vi "Rename Node Name.vi"(8 "error in (no error)":errorcluster, 10 "Node Tag":string, 11 "TREE in":refnum<class "MyTreeAPI.lvclass">) -> (0 "error out":errorcluster, 3 "TREE out":refnum<class "MyTreeAPI.lvclass">)   [LabVIEW 2015, in "MyTreeAPI.lvclass"]
uses:
  MyTreeAPI.lvclass
  MyTreeAPI.lvclass/MyTreeAPI.ctl
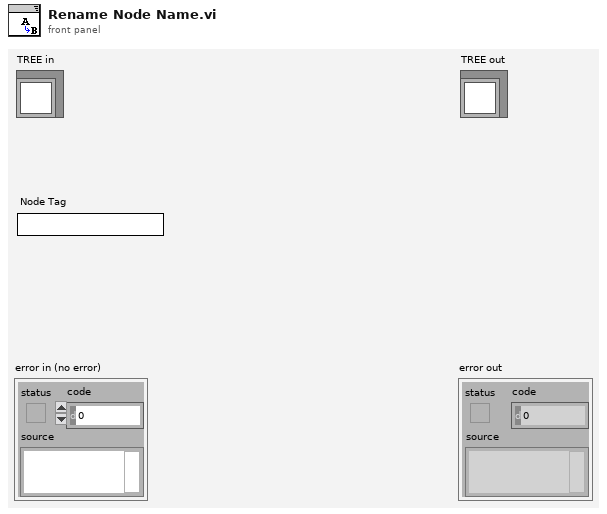
[diagram p1: front panel]
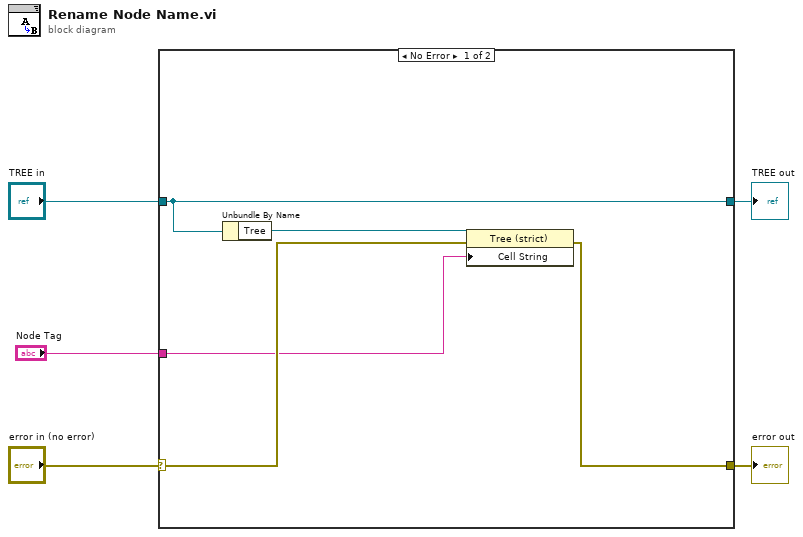
[diagram p0: block diagram]
diagram:
  n1 = case shown="No Error" "error in (no error)" {
    selector: "error in (no error)" -> [w8 w12]
    tunnel: [w6 w12] -> w4
    tunnel: [w10 w11] -> w2
    tunnel: "TREE in" -> [w10 w11]
    tunnel: "Node Tag" -> [w7 _]
    frame No Error {
      n2 = Unbundle By Name(w10) -> ("Tree"=w9:refnum<vi>)
      n3 = property class="Tree (strict)"(reference=w9, error in=w8, "Cell String"=w7) -> (error out=w6:errorcluster)  [unwired: 1 out]
    }
    frame Error {
    }
  }
  "error out" <- w4
  "TREE out" <- w2
